vi "Set Ignition Data.vi"(8 "error in":errorcluster, 10 "Tester Tx":T1, 11 "Sequence Context":refnum<k7>) -> (0 "error out":errorcluster, 3 "Tester Tx out":T1)   [LabVIEW 2019, in "Ignition.lvlib"]
uses:
  Ignition.lvlib
  <vilib>/addons/TestStand/_TSUtility.llb/TestStand - Get Property Value (String).vi
  <vilib>/addons/TestStand/_TSUtility.llb/TestStand - Get Property Value (Number {Signed 32-bit Integer}).vi
  <vilib>/addons/TestStand/_TSUtility.llb/TestStand - Get Property Value (Number {Unsigned 32-bit Integer}).vi
  <vilib>/addons/TestStand/_TSUtility.llb/TestStand - Get Property Value (Numeric Array).vi
  Tester Tx.ctl
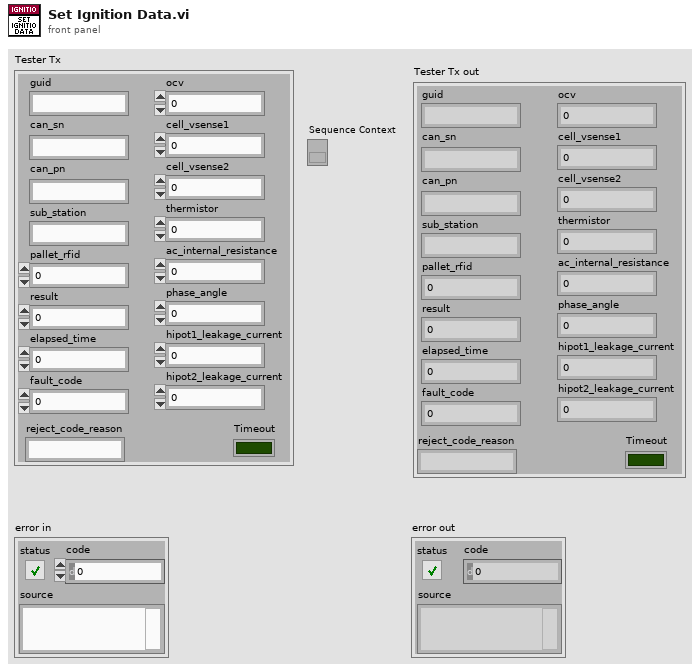
[diagram p1: front panel]
types:
  T1 = typedef "Ignition.lvlib/Tester Tx.ctl" = cluster{"thermistor":dbl, "phase_angle":dbl, "pallet_rfid":dbl, "ocv":dbl, "cell_vsense1":dbl, "cell_vsense2":dbl, "hipot1_leakage_current":dbl, "hipot2_leakage_current":dbl, "guid":string, "can_sn":string, "can_pn":string, "ac_internal_resistance":dbl, "sub_station":string, "fault_code":i32, "elapsed_time":i32, "result":i32, "reject_code_reason":string, "Timeout":bool}
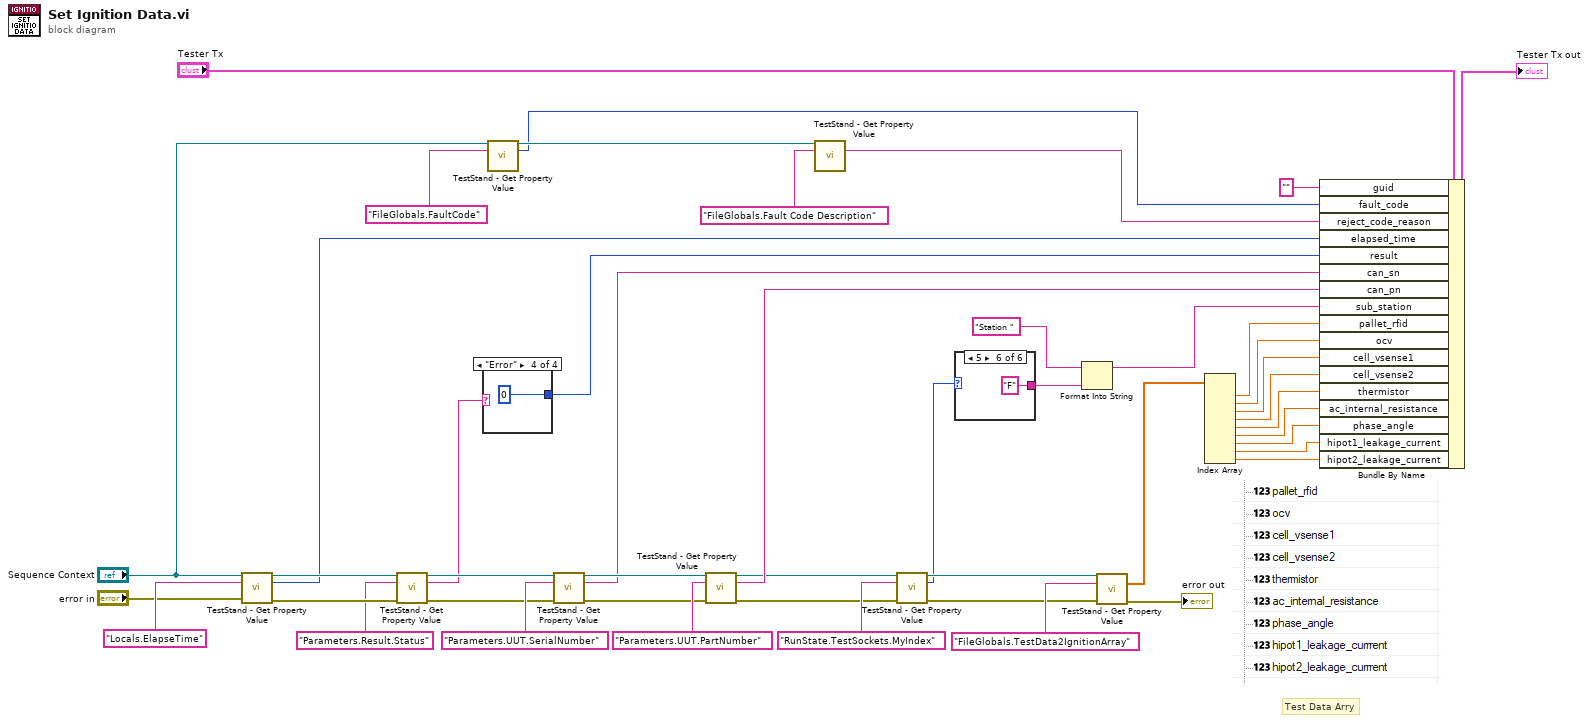
[diagram p0: block diagram]
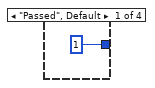
[diagram p2: hidden frame]
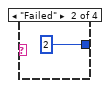
[diagram p3: hidden frame]
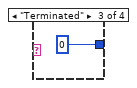
[diagram p4: hidden frame]
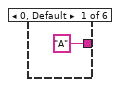
[diagram p5: hidden frame]
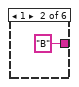
[diagram p6: hidden frame]
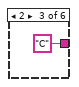
[diagram p7: hidden frame]
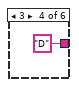
[diagram p8: hidden frame]
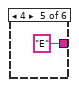
[diagram p9: hidden frame]
diagram:
  # "Test Data Arry"
  n1 = call-poly <vilib>:"TestStand - Get Property Value.vi"("Sequence Context In"="Sequence Context", "Lookup String"="Locals.ElapseTime", "error in (no error)"="error in") -> ("Sequence Context Out"=w17:refnum<k7>, "Value"=w13:i32, "error out"=w19:errorcluster)  [unwired: 10 in]
  n2 = call-poly <vilib>:"TestStand - Get Property Value.vi"("Sequence Context In"=w17, "Lookup String"="Parameters.Result.Status", "error in (no error)"=w19) -> ("Sequence Context Out"=w16:refnum<k7>, "Value"=w12:string, "error out"=w15:errorcluster)  [unwired: 10 in]
  n3 = case shown="\"Error\"" w12 {
    tunnel: [1 2 0 0] -> w11
    frame "Passed", Default {
    }
    frame "Failed" {
    }
    frame "Terminated" {
    }
    frame "Error" {
    }
  }
  n4 = call-poly <vilib>:"TestStand - Get Property Value.vi"("Sequence Context In"="Sequence Context", "Lookup String"="FileGlobals.FaultCode") -> ("Sequence Context Out"=w4:refnum<k7>, "Value"=w1:i32)  [unwired: 11 in, 1 out]
  n5 = call-poly <vilib>:"TestStand - Get Property Value.vi"("Sequence Context In"=w16, "Lookup String"="Parameters.UUT.SerialNumber", "error in (no error)"=w15) -> ("Sequence Context Out"=w45:refnum<k7>, "Value"=w42:string, "error out"=w43:errorcluster)  [unwired: 10 in]
  n6 = call-poly <vilib>:"TestStand - Get Property Value.vi"("Sequence Context In"=w45, "Lookup String"="Parameters.UUT.PartNumber", "error in (no error)"=w43) -> ("Sequence Context Out"=w23:refnum<k7>, "Value"=w41:string, "error out"=w39:errorcluster)  [unwired: 10 in]
  n7 = call-poly <vilib>:"TestStand - Get Property Value.vi"("Sequence Context In"=w4, "Lookup String"="FileGlobals.Fault Code Description") -> ("Value"=w2:string)  [unwired: 11 in, 2 out]
  n8 = call-poly <vilib>:"TestStand - Get Property Value.vi"("Sequence Context In"=w23, "Lookup String"="RunState.TestSockets.MyIndex", "error in (no error)"=w39) -> ("Sequence Context Out"=w37:refnum<k7>, "Value"=w22:u32, "error out"=w35:errorcluster)  [unwired: 10 in]
  n9 = case shown="5" w22 {
    tunnel: ["A" ("format string") "B" ("format string") "C" ("format string") "D" ("format string") "E" ("format string") "F" ("format string")] -> w21
    frame 0, Default {
    }
    frame 1 {
    }
    frame 2 {
    }
    frame 3 {
    }
    frame 4 {
    }
    frame 5 {
    }
  }
  n10 = Format Into String(initial string="Station ", w21) -> (resulting string=w38:string)  [unwired: 2 in, 1 out]
  n11 = call-poly <vilib>:"TestStand - Get Property Value.vi"("Sequence Context In"=w37, "Lookup String"="FileGlobals.TestData2IgnitionArray", "error in (no error)"=w35) -> ("Value"=w34:dbl[], "error out"=→"error out":errorcluster)  [unwired: 10 in, 1 out]
  n12 = Index Array(array=w34) -> (element #1=w33:dbl, element #2=w32:dbl, element #3=w31:dbl, element #4=w30:dbl, element #5=w29:dbl, element #6=w28:dbl, element #7=w27:dbl, element #8=w26:dbl, element #9=w25:dbl)  [unwired: 9 in]
  n13 = Bundle By Name(cluster="Tester Tx", "guid"="", "fault_code"=w1, "reject_code_reason"=w2, "elapsed_time"=w13, "result"=w11, "can_sn"=w42, "can_pn"=w41, "sub_station"=w38, "pallet_rfid"=w33, "ocv"=w32, "cell_vsense1"=w31, "cell_vsense2"=w30, "thermistor"=w29, "ac_internal_resistance"=w28, "phase_angle"=w27, "hipot1_leakage_current"=w26, "hipot2_leakage_current"=w25) -> (→"Tester Tx out":T1)
